vi "OneSessTwoPinOneInstrOneSiteReservation_CallNiScopeGetConnections1PinMConnections_ReturnsTwoConnections.vi"(8 "error in":errorcluster) -> (0 "error out":errorcluster, 2 "result":string, 3 "pass":bool)   [LabVIEW 2020, in "MeasurementServerTests.lvlib"]
uses:
  MeasurementServerTests.lvlib
  Runtime/MeasurementLink Session Management/Session Reservation/Connection.ctl
  Runtime/MeasurementLink niScope/Connection with Session.ctl
  a536e905-e99b-4ce6-9f7b-add65bd26abc.vi
  03fc85e1-696b-4ece-a78b-f41470766ac0.vi
  b3e5c3be-b7a7-4b6e-86ee-709eea9cb752.vi
  Runtime/MeasurementLink Session Management/Session Reservation/Session Reservation.lvclass
  Runtime/MeasurementLink niScope/MeasurementLink niScope.lvlib
  Runtime/MeasurementLink niScope/Get Connections - 1Pin MConn.vi
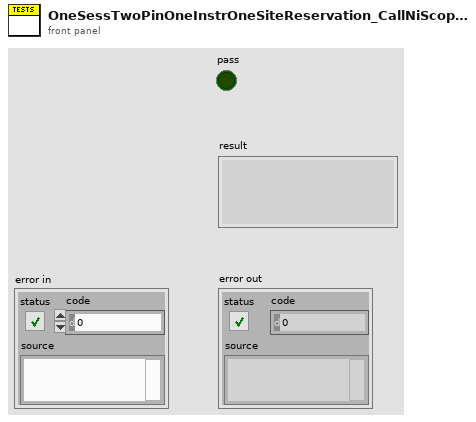
[diagram p1: front panel]
types:
  T1 = typedef "MeasurementLink Session Management.lvlib/Session Reservation.lvclass/Connection.ctl" = cluster{"pin or relay name":string, "site":i32, "instrument type id":string, "channel":string}
  T2 = typedef "MeasurementLink niScope.lvlib/Connection with Session.ctl" = cluster{"connection":T1, "session":refnum<k15>}
  T3 = typedef "MeasurementLink Session Management.lvlib/Session Reservation.lvclass/Data.ctl" = cluster{"session and driver infos":T4[], "pin or relay names":string[]}
  T4 = typedef "MeasurementLink Session Management.lvlib/Session Reservation.lvclass/Session and Driver Info.ctl" = cluster{"session info":T5, "session":variant}
  T5 = typedef "MeasurementLink Session Management Client.lvlib/ni_measurementlink_sessionmanagement_v1_SessionInformation.ctl" = cluster{"session":T6, "resource_name":string, "channel_list":string, "instrument_type_id":string, "session_exists":bool, "channel_mappings":T7[]}
  T6 = typedef "MeasurementLink Session Management Client.lvlib/nidevice_grpc_Session.ctl" = cluster{"name":string}
  T7 = typedef "MeasurementLink Session Management Client.lvlib/ni_measurementlink_sessionmanagement_v1_ChannelMapping.ctl" = cluster{"pin_or_relay_name":string, "site":i32, "channel":string}
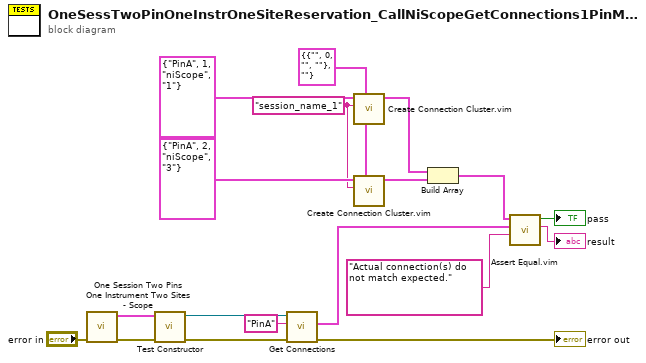
[diagram p0: block diagram]
diagram:
  w5 = T2 {"connection"={"pin or relay name"="", "site"=0, "instrument type id"="", "channel"=""}, "session"=""} ("niDCPower connection")
  w4 = "session_name_1" ("session in")
  n1 = call "One Session Two Pins One Instrument Two Sites - Scope.vi"("error in"="error in") -> ("error out"=w11:errorcluster, "data out"=w10:T3)  [unwired: 9 in]
  n2 = call "Test Constructor.vi"("error in"=w11, "data"=w10) -> ("error out"=w18:errorcluster, "Session Reservation out"=w17:refnum<class "Session Reservation.lvclass">)  [unwired: 8 in]
  n3 = call-poly "Get Connections.vi"("error in"=w18, "pin or relay name"="PinA", "session reservation in"=w17) -> ("error out"=→"error out":errorcluster, "connections"=w15:T2[])  [unwired: 6 in, 1 out]
  n4 = call "Create Connection Cluster.vim"("connection type"=w5, "session in"=w4, "hardware independent connection in"=T1 {"pin or relay name"="PinA", "site"=1, "instrument type id"="niScope", "channel"="1"} ("connection")) -> ("connection out"=w3:T2)  [unwired: 8 in]
  n5 = call "Create Connection Cluster.vim"("connection type"=w5, "session in"=w4, "hardware independent connection in"=T1 {"pin or relay name"="PinA", "site"=2, "instrument type id"="niScope", "channel"="3"} ("connection")) -> ("connection out"=w2:T2)  [unwired: 8 in]
  n6 = Build Array(w3, w2) -> (w1:T2[])
  n7 = call "Assert Equal.vim"("failure message"="Actual connection(s) do not match expected.", "actual value"=w15, "expected value"=w1) -> ("message"=→"result":string, "equal?"=→"pass":bool)  [unwired: 7 in]
